vi "PQparamtype.vi"(7 "error in (no error)":errorcluster, 9 "param_num":u64, 10 "res":u64) -> (0 "error out":errorcluster, 2 "PQparamtype":u64, 3 "res_out":u64)   [LabVIEW 2019, in "libpqlv64.lvlib"]
uses:
  libpqlv64.lvlib
  libpq.dll
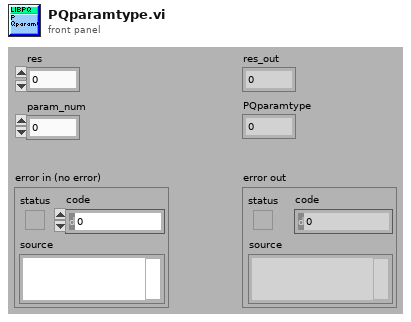
[diagram p1: front panel]
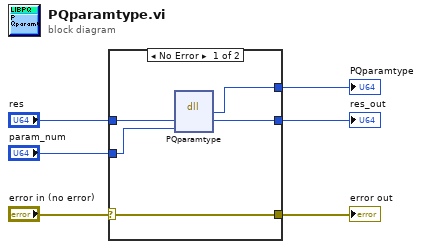
[diagram p0: block diagram]
diagram:
  n1 = case shown="No Error" "error in (no error)" {
    selector: "error in (no error)" -> [w11 w13]
    tunnel: [w11 w13] -> w5
    tunnel: [w10 _] -> w4
    tunnel: "param_num" -> [w9 _]
    tunnel: "res" -> [w8 w12]
    tunnel: [w7 w12] -> w1
    frame No Error {
      n2 = dll-call lib="libpq.*" fn="PQparamtype"("res"=w8, "param_num"=w9) -> ("PQparamtype"=w10:u64, "res"=w7:u64)  [unwired: 4 in, 2 out]
    }
    frame Error {
    }
  }
  "PQparamtype" <- w4
  "error out" <- w5
  "res_out" <- w1
